vi "Period and Phase Measurement.vi"() -> ()   [LabVIEW 2018]
doc: "This VI Simulates two signals at the same frequency and a user defined phase offset. These simulated inputs are then used to demonstrate the phase and measurement capability of the example. A Single Cycle Timed Loop is used."
uses:
  <vilib>/Platform/TimedLoop/XDataNode/timing_clust.ctl
  <vilib>/Platform/TimedLoop/XDataNode/nitl_modes.ctl
  <vilib>/Platform/TimedLoop/XDataNode/wakeup.ctl
  <vilib>/rvi/Emulation/niFpgaGetClockAttributes.vi
  <vilib>/rvi/Emulation/niFpgaSctlEmulationGetInTimedLoop.vi
  <vilib>/rvi/Emulation/niFpgaEmulationReportErrorSimple.vi
  <vilib>/rvi/Emulation/niFpgaProcessEmulError.vi
  <vilib>/rvi/Emulation/niFpgaCriticalErrorInLSC.vi
  <vilib>/Platform/TimedLoop/XDataNode/XDataNode.xnode
  <vilib>/Platform/TimedLoop/XDataNode/XDNodeRunTimeDep.lvlib
panel:
  out "Measured Period (Ticks)":u32
  out "Measured Phase Shift (Ticks)":u32
  out "Digital Signal B":bool
  in  "Period (mSec)":u32=40 caption="Count(uSec)"
  in  "Phase Shift (Deg)":u8=180 caption="Count(uSec)" max=180
  out "Digital Signal A":bool
  # "Overview: Demonstrates Period and Phase Measurement on an FPGA\nRequirements: LabVIEW FPGA\nInstructions:\n1. Run the VI\n2. Toggle Period to change the frequency of Signal A and Signal B\n3. Toggle Phase Shift to change the phase between Signal A and Signal B"
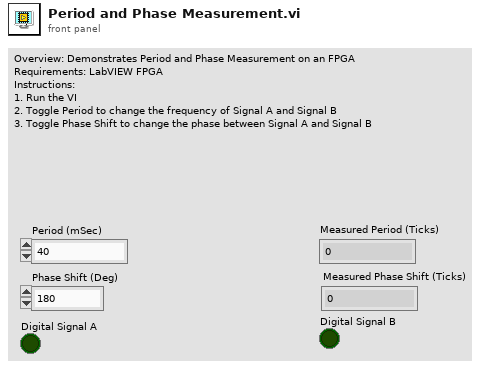
[diagram p1: front panel]
types:
  T1 = typedef "XDNodeRunTimeDep.lvlib/timing_clust.ctl" = cluster{"Expected End [f-1]":u64, "Actual End [f-1]":u64, "Finished Late? [f-1]":bool, "Expected End [i-1]":u64, "Actual End [i-1]":u64, "Finished Late? [i-1]":bool, "Expected Start [i]":u64, "Actual Start [i]":u64, "Expected Start [f]":u64, "Actual Start [f]":u64, "Source Name":string, "Structure Name":string, "Period":i64, "Deadline":i64, "Offset":i64, "Start":i64, "Priority":i32, "Timeout":i32, "Mode":T2, "Wakeup Reason":T3, "Error":errorcluster, "Source Type":string, "Secondary Source Type":string, "Global End Time":u64, "Global Start Time":u64, "Frame Duration":u64, "Iteration Duration":u64, "Assigned CPU":i32, "I/O Scan Engine Mode":u32}
  T2 = typedef "XDNodeRunTimeDep.lvlib/nitl_modes.ctl" = enum32{"No Change", "Process missed periods, maintain original phase", "Discard missed periods, maintain original phase", "Process missed periods, ignore original phase", "Discard missed periods, ignore original phase"}
  T3 = typedef "XDNodeRunTimeDep.lvlib/wakeup.ctl" = enum32{"Normal", "Aborted", "Asynchronous wakeup", "Timing source error", "Timed loop error", "Timeout"}
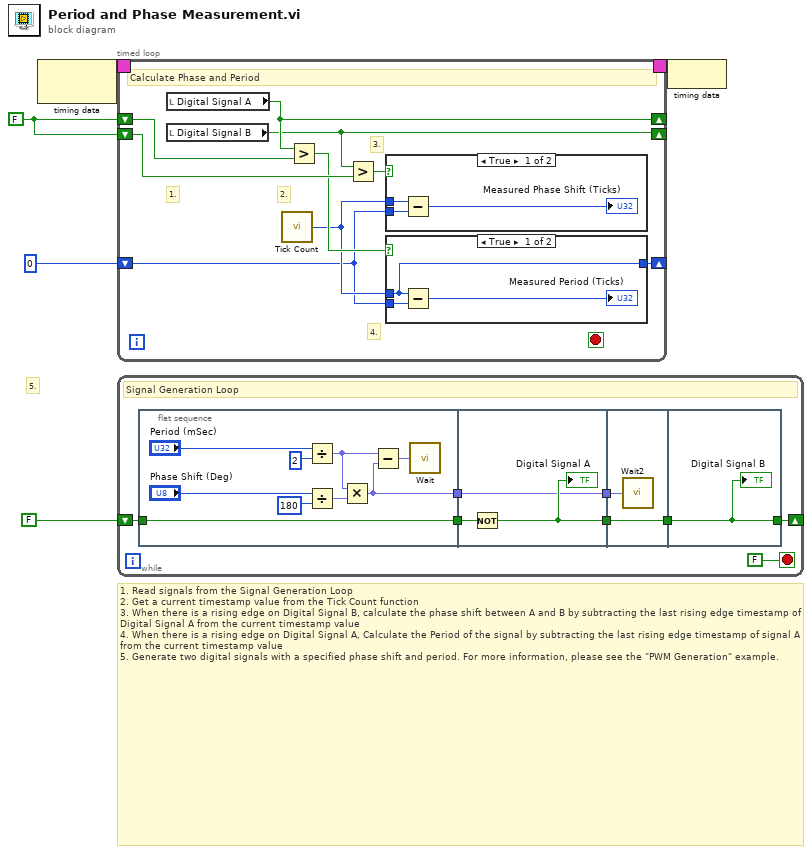
[diagram p0: block diagram]
diagram:
  w2 = FALSE ("Digital Signal A")
  # "5."
  # "1. Read signals from the Signal Generation Loop\n2. Get a current timestamp value from the Tick Count function\n3. When there is a rising edge on Digital Signal B, calculate the phase shift between A and B by subtracting the last rising edge timestamp of Digital Signal A from the current timestamp value\n4. When there is a rising edge on Digital Signal A, Calculate the Period of the signal by subtracting the last rising edge timestamp of signal A from the current timestamp value\n5. Generate two digital signals with a specified phase shift and period. For more information, please see the \"PWM Generation\" example."
  n1 = node-c288() -> (w5:T1)  [unwired: 1 in]
  n2 = timed-loop "Two Edge Separation" {
    shift-left: w2 -> [w13]
    shift-right: [w11] -> _
    shift-left: u32 0 ("Tick Count(Ticks)") -> [w7]
    shift-right: [w6] -> _
    shift-left: w2 -> [w14]
    shift-right: [w12] -> _
    timing: w5 -> [_]
    timing-out: [_] -> w4
    stop <- _ stop-if-true
    # "4."
    # "3."
    # "2."
    # "1."
    # "Calculate Phase and Period"
    n3 = local read "Digital Signal A"() -> (w12:bool)
    n4 = local read "Digital Signal B"() -> (w11:bool)
    n5 = call "Tick Count"() -> ("Tick Count(Ticks)"=w8:u32)
    n6 = Greater?(x=w12, y=w14) -> (0:w9:bool)
    n7 = Greater?(x=w11, y=w13) -> (0:w10:bool)
    n8 = case shown="True" w10 {
      tunnel: w8 -> [w20 _]
      tunnel: w7 -> [w21 _]
      frame True {
        n9 = Subtract(x=w20, y=w21) -> (x-y=→"Measured Phase Shift (Ticks)":u32)
      }
      frame False {
      }
    }
    n10 = case shown="True" w9 {
      tunnel: w8 -> [w15 _]
      tunnel: w7 -> [w16 w18]
      tunnel: [w15 w18] -> w6
      frame True {
        n11 = Subtract(x=w15, y=w16) -> (x-y=→"Measured Period (Ticks)":u32)
      }
      frame False {
      }
    }
  }
  n12 = while {
    shift-right: [w31] -> _
    shift-left: FALSE -> [w26]
    stop <- FALSE stop-if-true
    # "Signal Generation Loop"
    n13 = flat-sequence {
      tunnel: [w36] -> w27
      tunnel: w26 -> [w32]
      tunnel: [w32] -> w25
      tunnel: [w43] -> w30
      tunnel: [w42] -> w28
      tunnel: w27 -> [w42]
      tunnel: w25 -> [w41]
      tunnel: w30 -> [w45]
      tunnel: [w45] -> w29
      tunnel: w28 -> [w44]
      tunnel: [w46] -> w31
      tunnel: w29 -> [w46]
      frame #0 {
        n14 = Divide(x="Period (mSec)", y=u32 2) -> (x/y=w33:fxp<+/-,32,26>)
        n15 = Divide(x="Phase Shift (Deg)", y=u32 180) -> (x/y=w38:fxp<+/-,32,16>)
        n16 = Multiply(x=w33, y=w38) -> (x*y=w36:fxp<+/-,64,42>)
        n17 = Subtract(x=w33, y=w36) -> (x-y=w37:fxp<+/-,64,42>)
        n18 = call "Wait"("Count(mSec)"=w37) -> ()  [unwired: 1 out]
      }
      frame #1 {
        n19 = Not(x=w41) -> (.not. x?=w43:bool)
        "Digital Signal A" <- w43
      }
      frame #2 {
        n20 = call "Wait2"("Count(mSec)"=w44) -> ()  [unwired: 1 out]
      }
      frame #3 {
        "Digital Signal B" <- w46
      }
    }
  }
  n21 = node-c288(w4) -> ()
